vi "running_avg.vi"(2 "Size of data":i32=10 caption="Size of data (10)", 3 "New value":dbl caption="New value (0)", 4 "Speed in ms":i32=250 caption="Speed in ms (250)") -> (0 "Data":dbl[](array[numeric]), 1 "Running average":dbl format="%0.2f")   [LabVIEW 2016]
doc: "The Running Average VI calculates a running average of an array with dynamic length and dynamic sampling speed. The VI allocates values to the <b>Data</b> array. The <b>Size of data</b> control determines the array length. When the VI reaches the last index of <b>Data</b>, the process begins again at the zero index. During each while loop iteration, the VI complies the sum of all elements in <b>Data</b> and divides that value by the length of the <b>Data</b> array, determining the running average with dynamic length and speed. The VI displays the value of <b>Running average</b> for each while loop iteration."
uses:
  <vilib>/Analysis/baseanly.llb/Mean (DBL).vi
  <vilib>/Analysis/NI_AALBase.lvlib
panel:
  in  "stop":bool
  # "Select Help»Show Context Help and move the cursor \nover the VI icon to display help for this VI."
  # "Instructions:\n\n1)  Run VI\n2)  Adjust the value of the New value control\n3)  Observe the Running average indicator and the Data array.\n4)  Click the Stop button.\n5)  Adjust the Size of data and Speed in ms controls and run VI again to return new results."
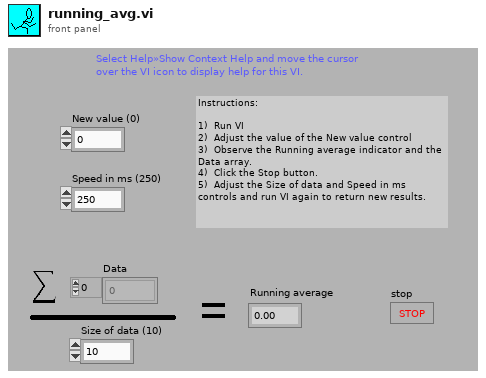
[diagram p1: front panel]
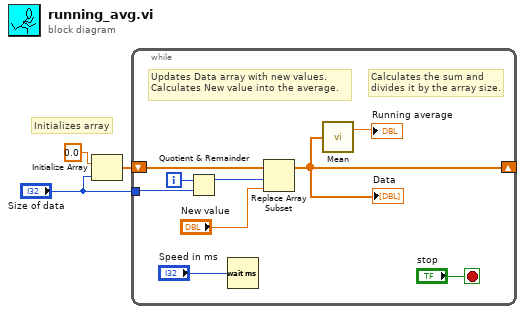
[diagram p0: block diagram]
diagram:
  # "Initializes array"
  n1 = Initialize Array(0.0 ("element"), "Size of data") -> (w2:dbl[])
  n2 = while {
    shift-right: [w5] -> _
    shift-left: w2 -> [w8]
    tunnel: "Size of data" -> [w7]
    i -> [w10]
    stop <- "stop" stop-if-true
    # "Updates Data array with new values.\nCalculates New value into the average."
    # "Calculates the sum and divides it by the array size."
    n3 = Quotient & Remainder(x=w10, y=w7) -> (x-y*floor(x/y)=w11:i32)  [unwired: 1 out]
    n4 = Wait (ms)(milliseconds to wait="Speed in ms") -> ()  [unwired: 1 out]
    n5 = Replace Array Subset(array=w8, new element="New value", index=w11) -> (w5:dbl[])
    "Data" <- w5
    n6 = call-poly <vilib>:"Mean.vi"("X"=w5) -> ("mean"=→"Running average":dbl)  [unwired: 1 out]
  }
